vi "sub_HOSTTOFPGA Voltage.vi"(1 "Input":dbl) -> (0 "Output":i16)   [LabVIEW 2015]
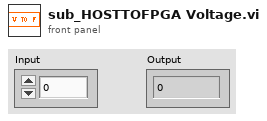
[diagram p1: front panel]
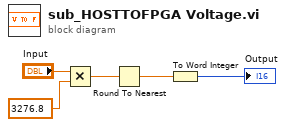
[diagram p0: block diagram]
diagram:
  n1 = Multiply(x="Input", y=3276.8) -> (x*y=w3:dbl)
  n2 = Round To Nearest(number=w3) -> (nearest integer value=w1:dbl)
  n3 = To Word Integer(number=w1) -> (16bit integer=→"Output":i16)
